vi "read_protocol_json.vi"(11 "Path":path) -> (0 "stims":path[](array[path]), 1 "n_stims":i32, 2 "rate":i32, 3 "protocol name":string, 4 "error out":errorcluster)   [LabVIEW 2015]
panel:
  out "JSON Out":string[](array[string])
  out "JSON text":string
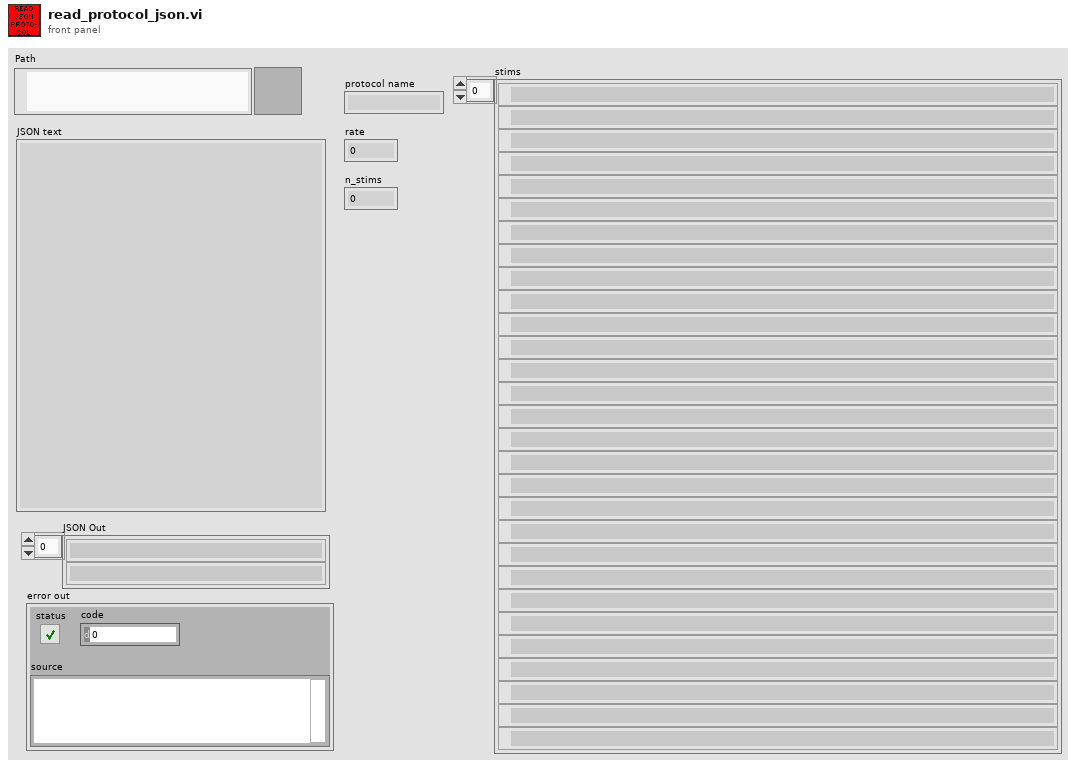
[diagram p1: front panel]
types:
  T1 = enum16{"open", "replace", "create", "open or create", "replace or create", "replace or create with confirmation"}
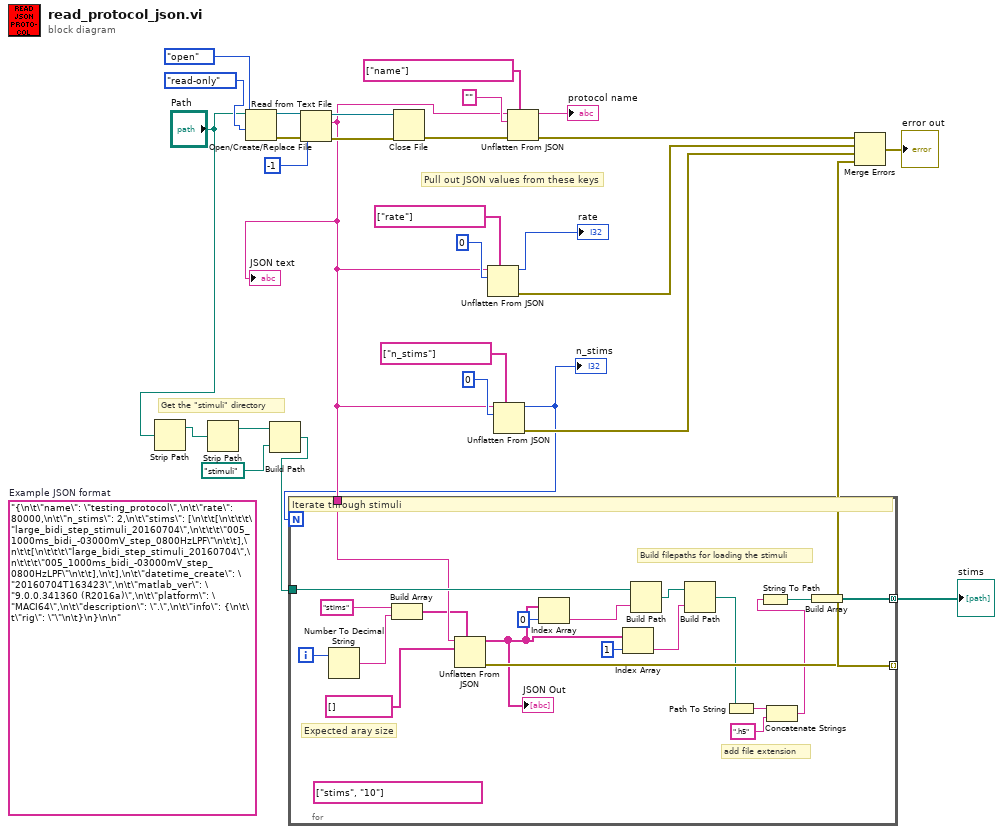
[diagram p0: block diagram]
diagram:
  (unwired) "{\n\t\"name\": \"testing_protocol\",\n\t\"rate\": 80000,\n\t\"n_stims\": 2,\n\t\"stims\": [\n\t\t[\n\t\t\t\"large_bidi_step_stimuli_20160704\",\n\t\t\t\"005_1000ms_bidi_-03000mV_step_0800HzLPF\"\n\t\t],\n\t\t[\n\t\t\t\"large_bidi_step_stimuli_20160704\",\n\t\t\t\"005_1000ms_bidi_-03000mV_step_0800HzLPF\"\n\t\t],\n\t],\n\t\"datetime_create\": \"20160704T163423\",\n\t\"matlab_ver\": \"9.0.0.341360 (R2016a)\",\n\t\"platform\": \"MACI64\",\n\t\"description\": \".\",\n\t\"info\": {\n\t\t\"rig\": \"\"\n\t}\n}\n\n"  # Example JSON format
  # "Pull out JSON values from these keys"
  # "Get the \"stimuli\" directory"
  n1 = Strip Path(path="Path") -> (stripped path=w6:path)  [unwired: 1 out]
  n2 = Strip Path(path=w6) -> (stripped path=w5:path)  [unwired: 1 out]
  n3 = Open/Create/Replace File(file path (use dialog)="Path", operation (0:open)=T1."open", access (0:read/write)=enum16{"read/write", "read-only", "write-only"}."read-only") -> (refnum out=w26:refnum<file>, error out=w25:errorcluster)  [unwired: 3 in, 1 out]
  n4 = Build Path(base path=w5, name or relative path=path "stimuli") -> (appended path=w2:path)
  n5 = Read from Text File(file (use dialog)=w26, count=-1, error in=w25) -> (refnum out=w28:refnum<file>, text=w10:string, error out=w27:errorcluster)  [unwired: 1 in, 1 out]
  "JSON text" <- w10
  n6 = Close File(refnum=w28, error in=w27) -> (error out=w22:errorcluster)  [unwired: 1 out]
  n7 = Unflatten From JSON(path=string[] ["rate"], JSON string=w10, type and defaults=0) -> (value=→"rate":i32, error out=w13:errorcluster)  [unwired: 4 in]
  n8 = Unflatten From JSON(path=string[] ["n_stims"], JSON string=w10, type and defaults=0) -> (value=w3:i32, error out=w9:errorcluster)  [unwired: 4 in]
  "n_stims" <- w3
  n9 = for {
    N: w3 -> [_]
    tunnel: w10 -> [w43]
    tunnel: [w47] -> w8 mode=indexing
    tunnel: w2 -> [w46]
    tunnel: [w45] -> w1 mode=concatenating
    i -> [w48]
    (unwired) string[] ["stims", "10"]
    # "add file extension"
    # "Expected aray size"
    # "Build filepaths for loading the stimuli"
    # "Iterate through stimuli"
    n10 = Number To Decimal String(number=w48) -> (decimal integer string=w41:string)  [unwired: 1 in]
    n11 = Build Array("stims", w41) -> (w40:string[])
    n12 = Unflatten From JSON(path=w40, JSON string=w43, type and defaults=string[] []) -> (value=w36:string[], error out=w47:errorcluster)  [unwired: 4 in]
    "JSON Out" <- w36
    n13 = Index Array(array=w36, index=0) -> (element=w38:string)
    n14 = Index Array(array=w36, index=1) -> (element=w35:string)
    n15 = Build Path(base path=w46, name or relative path=w38) -> (appended path=w44:path)
    n16 = Build Path(base path=w44, name or relative path=w35) -> (appended path=w34:path)
    n17 = Path To String(path=w34) -> (string=w33:string)
    n18 = Concatenate Strings(w33, ".h5") -> (w31:string)
    n19 = String To Path(string=w31) -> (path=w30:path)
    n20 = Build Array(w30) -> (w45:path[])
  }
  "stims" <- w1
  n21 = Unflatten From JSON(path=string[] ["name"], JSON string=w10, type and defaults="", error in (no error)=w22) -> (value=→"protocol name":string, error out=w15:errorcluster)  [unwired: 3 in]
  n22 = Merge Errors(w15, w13, w9, w8) -> (→"error out":errorcluster)
